vi "_PC_Pub_Write_Spreadsheet.vi"(6 "append to file? (new file:F)":bool, 7 "delimiter (\\t)":string="\t", 8 "error in (no error)":errorcluster, 9 "1D Data":string[](array[string]), 10 "2D Data":string[][](array[string]), 11 "file path (use dialog)":path) -> (0 "error out":errorcluster, 3 "Path out":path)   [LabVIEW 2018]
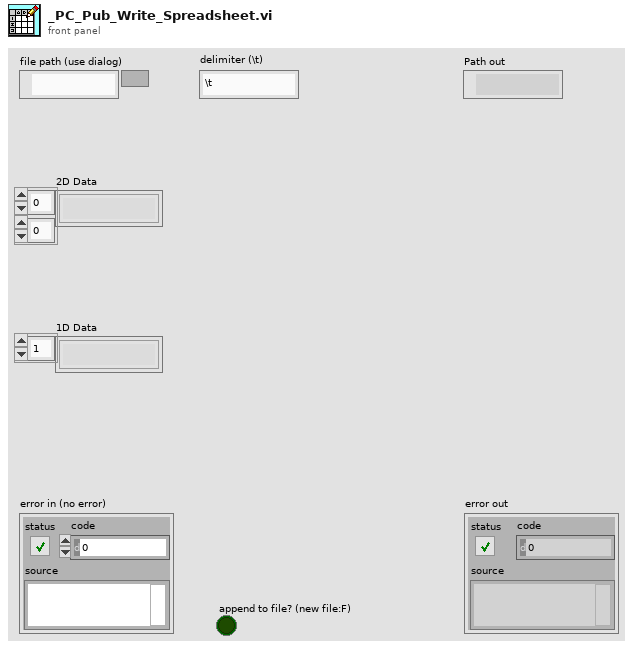
[diagram p1: front panel]
types:
  T1 = enum16{"open", "replace", "create", "open or create", "replace or create", "replace or create with confirmation"}
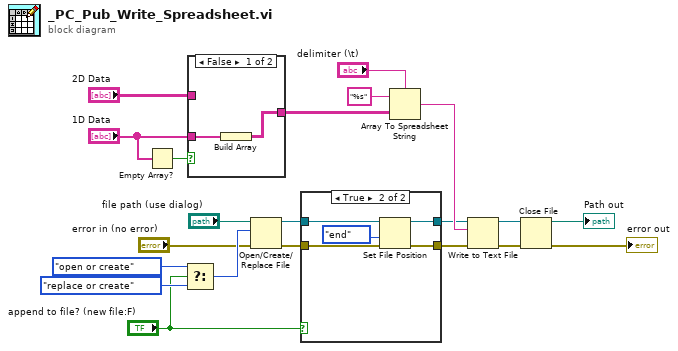
[diagram p0: block diagram]
diagram:
  n1 = Empty Array?(array="1D Data") -> (empty?=w4:bool)
  n2 = Select ("function")(t=T1."open or create" ("operation (0:open)"), s="append to file? (new file:F)", f=T1."replace or create" ("operation (0:open)")) -> (s? t:f=w13:T1)
  n3 = case shown="False" w4 {
    tunnel: "1D Data" -> [w23 _]
    tunnel: "2D Data" -> [_ w24]
    tunnel: [w22 w24] -> w1
    frame False {
      n4 = Build Array(w23) -> (w22:string[][])
    }
    frame True {
    }
  }
  n5 = Open/Create/Replace File(file path (use dialog)="file path (use dialog)", error in="error in (no error)", operation (0:open)=w13) -> (refnum out=w9:refnum<file>, error out=w8:errorcluster)  [unwired: 3 in, 1 out]
  n6 = case shown="True" "append to file? (new file:F)" {
    tunnel: w8 -> [w25 w31]
    tunnel: [w25 w30] -> w7
    tunnel: w9 -> [w26 w28]
    tunnel: [w26 w29] -> w6
    frame False {
    }
    frame True {
      n7 = Set File Position(refnum=w28, from (0:start)=enum16{"start", "end", "current"}."end", error in=w31) -> (refnum out=w29:refnum<file>, error out=w30:errorcluster)  [unwired: 1 in]
    }
  }
  n8 = Array To Spreadsheet String(delimiter (Tab)="delimiter (\\t)", array=w1, 3:"%s" ("format string")) -> (spreadsheet string=w20:string)
  n9 = Write to Text File(file (use dialog)=w6, text=w20, error in=w7) -> (refnum out=w19:refnum<file>, error out=w18:errorcluster)  [unwired: 1 in, 1 out]
  n10 = Close File(refnum=w19, error in=w18) -> (path=→"Path out":path, error out=→"error out":errorcluster)
